vi "Type_0.vi"(7 "프런트패널 윈도우:동작":T1(ring)=enum."Default", 8 "에러 입력":errorcluster caption="에러 입력(에러 없음)", 11 "세부분류코드":string caption="확장자없는 파일 이름") -> (0 "error out":errorcluster)   [LabVIEW 2020]
uses:
  Support/Controls/Cmd_Mouse Popup.ctl
  Support/Controls/Clst_Query Info.ctl
  Support/Controls/Cmd_Read Query.ctl
  Support/Public/Polymorph/Array Dedup_1D Str.vi
  Support/Public/Polymorph/Cell Space_Table.vi
  <vilib>/addons/database/NI_Database_API.lvlib
panel:
  in  "탭 컨트롤":enum32{"검색", "등록", "CMC"}(tab)
  in  "일부추가":bool
  out "인정범위":string[][](table)
  out "SQL Quary 컬럼명":string
  out "Calfunc":string[][](array[string])
  out "모델정보":string[][](array[string])
  in  "옵션검색":bool
  in  "옵션 검색 조건":string(combo)
  in  "모델검색":bool
  in  "모델 검색 조건":string
  in  "측정범위검색":bool
  in  "범위 검색 조건":dbl
  in  "전체추가":bool
  out "소분류코드":string
  out "측정기명":string
  in  "최대 측정 범위":i32(listbox)
  in  "모델 및 옵션 List":i32(listbox)
  out "Load Proc":string[][](table) caption="등록된 교정 Procedure"
  in  "교정기능":string(combo)
  in  "구분 2":string(combo) caption="측정방향"
  in  "참고 버튼":bool
  in  "교정값":string
  in  "명목값":string caption="명목값 (호칭)"
  in  "추가단위":string(combo)="mg" caption="단위"
  in  "구분":string(combo) caption="측정위치"
  out "Func_ext ?":bool
  out "배열":u32[](array[numeric])
  in  "단위":string(combo)
  in  "변경 버튼":bool
  in  "등록 버튼":bool
  in  "교정점 추가 버튼":bool
  in  "교정점":string
  in  "Proc":string[][](table) caption="등록할 교정 Procedure"
  in  "형식":string
  in  "옵션":string
  in  "최소눈금":string(combo)
  in  "교정기능 2":string(combo) caption="세부기능"
  in  "표시방식":string(combo)
  out "CMC":string[][](table)
  # "항목정보"
  # "검색옵션"
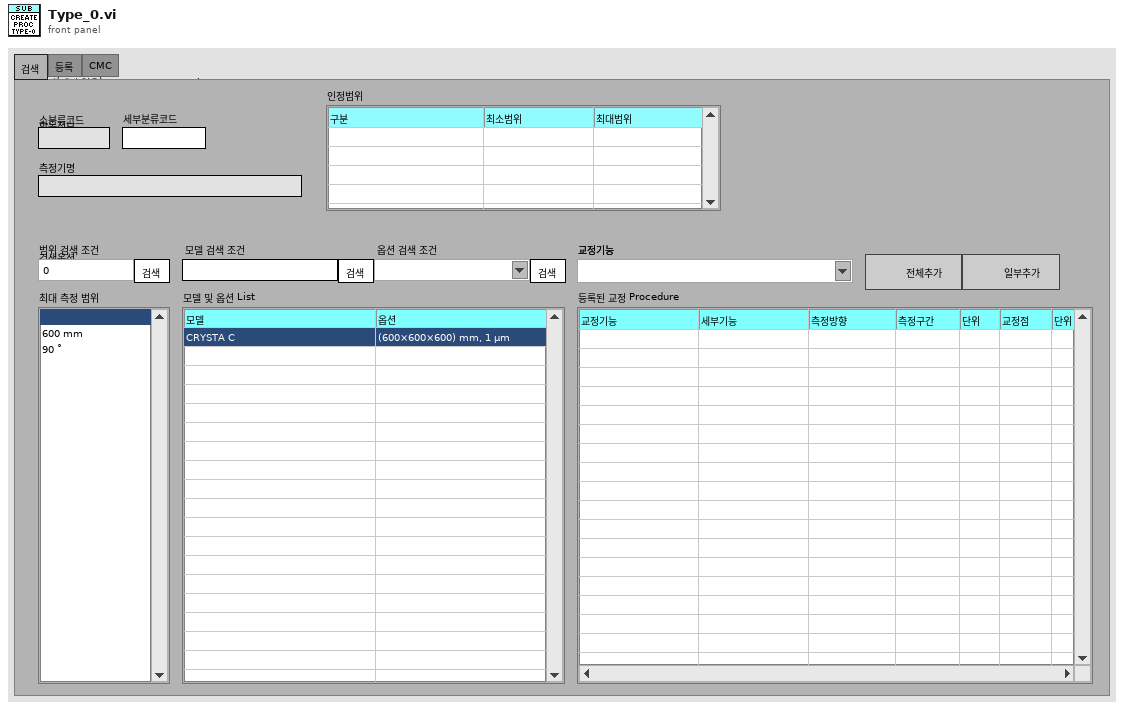
[diagram p1: front panel]
types:
  T1 = enum32{"Invalid", "Default", "Floating", "Floating/Auto-Hide", "Modal"}
  T2 = typedef "Cmd_Mouse Popup.ctl" = enum16{"활성화", "메뉴선택"}
  T3 = cluster{"Shift":bool, "Ctrl":bool, "Alt":bool, "Cmd":bool, "Opt":bool}
  T4 = typedef "Clst_Query Info.ctl" = cluster{"사번":string, "등록번호":string, "업체명":string, "세부분류코드":string, "형식":string, "기기번호":string, "FUNC":string, "FUNC_EXT":string, "옵션":string, "추가문자열":string, "일자":string, "배열 1":string[], "배열 2":string[], "항목명":string, "문자열":string, "이름":string}
  T5 = typedef "Cmd_Read Query.ctl" = enum16{"교정자 이름 얻기", "인증교정자 얻기", "기술책임자 얻기", "기책부책 얻기", "등록번호 얻기", "등록정보 얻기", "업체정보 얻기", "교정일자(CAMAS) 얻기", "교정일자(CALSTD) 얻기", "교정환경 얻기", "교정절차서 목록 얻기", "교정절차서명 얻기", "교정절차 목록얻기", "교정절차 얻기", "PROC 교정절차 얻기", "PROC SPEC 얻기", "교정절차(Func별) 얻기", "교정절차(Func_ext별) 얻기", "기관코드 얻기", "교정기능(세부분류) 얻기", "교정기능(모델) 얻기", "교정기능 목록 얻기", "교정기능 명칭 얻기", "교정기능 항목명칭 얻기", "DB (사용기준기) 얻기", "DB (기준기이름) 얻기", "DB (기준기이름목록) 얻기", "DB (기준기목록) 얻기", "DB (기준기값) 얻기", "DB (CMC) 얻기", "DB (FUNC) 얻기", "DB (CALNAME) 얻기", "DB (STDNAME) 얻기", "DB (SPEC) 얻기", "모델(항목전체) 얻기", "모델(최대범위) 얻기", "모델(최소범위) 얻기", "모델(최대최소) 얻기", "모델(범위조건) 얻기", "모델(등록요청) 얻기", "모델(형식별) 얻기", "모델(조건별) 얻기", "모델(모델검색) 얻기", "세부분류 목록 얻기", "기준기등록리스트 얻기", "STD Cal Date Check", "DB등록일자 얻기", "적용항목 얻기", "기타정보 얻기", "기준기요청 얻기", "서버버전 얻기"}
  T6 = cluster{refnum<vi>[], refnum<vi>[], refnum<vi>[], refnum<vi>[]}
  T7 = typedef "NI_Database_API.lvlib/Conn ObjectReference.ctl" = refnum<k1>
  T8 = typedef "LVRowAndColumnTypeDef.ctl" = cluster{"Row":i32, "Column":i32}
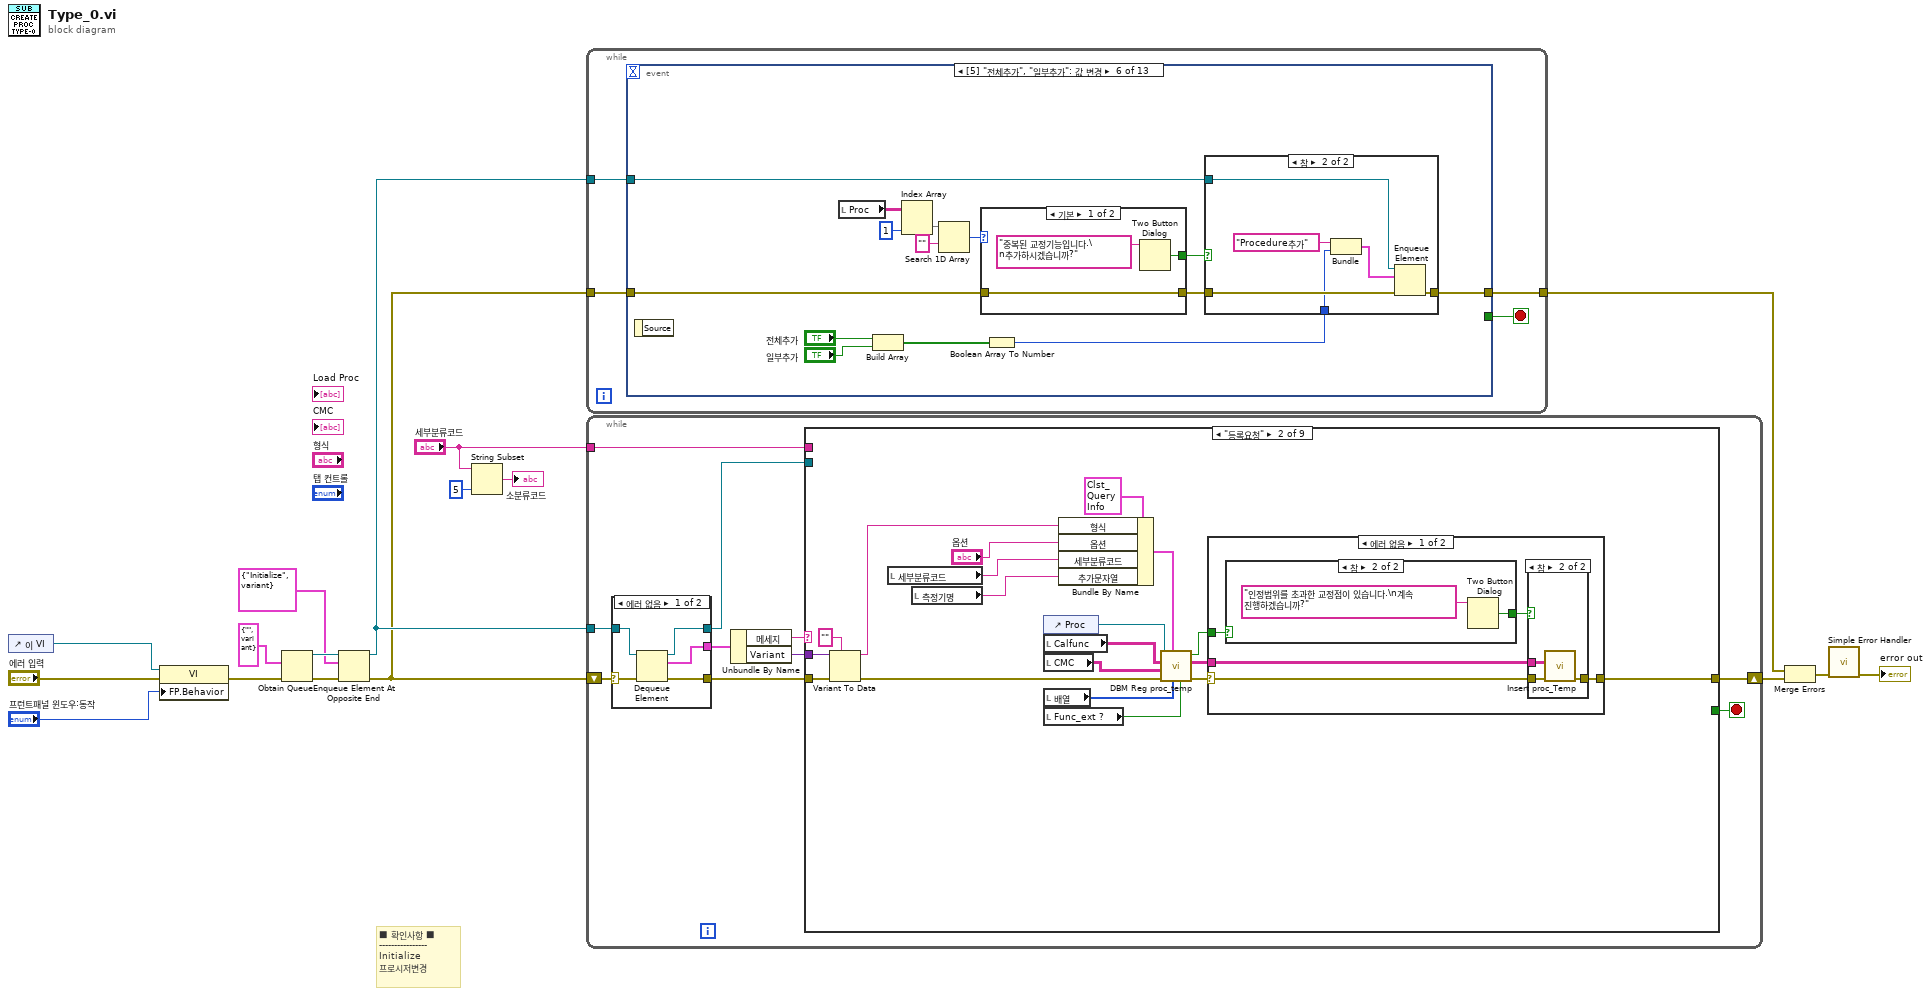
[diagram p0: block diagram]
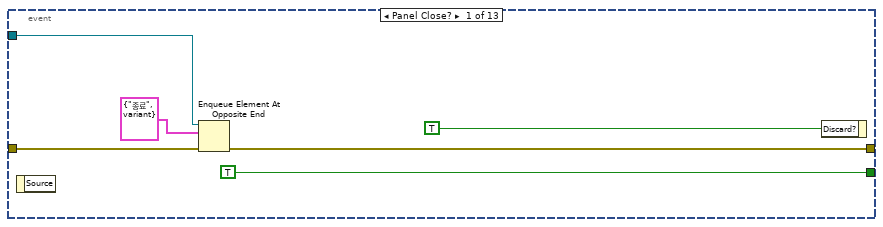
[diagram p2: hidden frame]
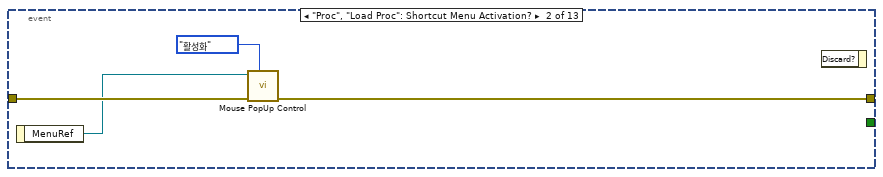
[diagram p3: hidden frame]
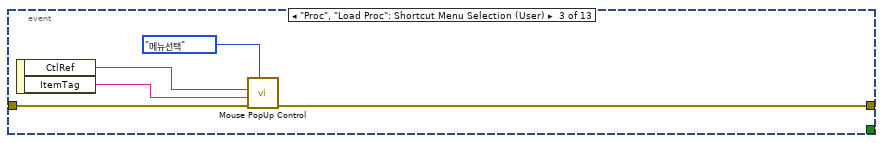
[diagram p4: hidden frame]
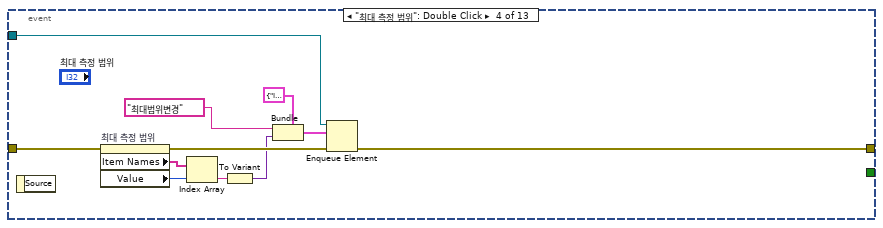
[diagram p5: hidden frame]
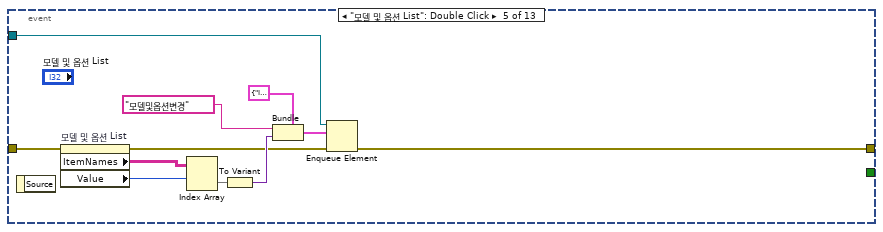
[diagram p6: hidden frame]
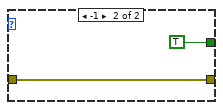
[diagram p8: hidden frame]
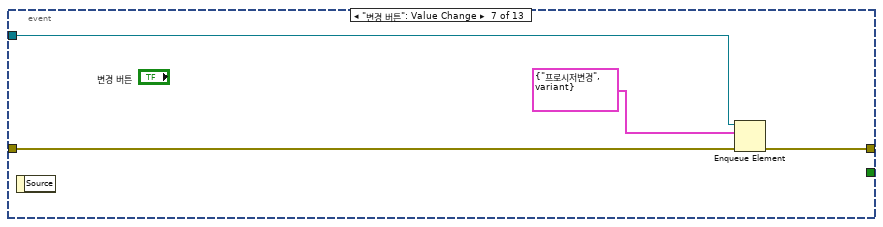
[diagram p9: hidden frame]
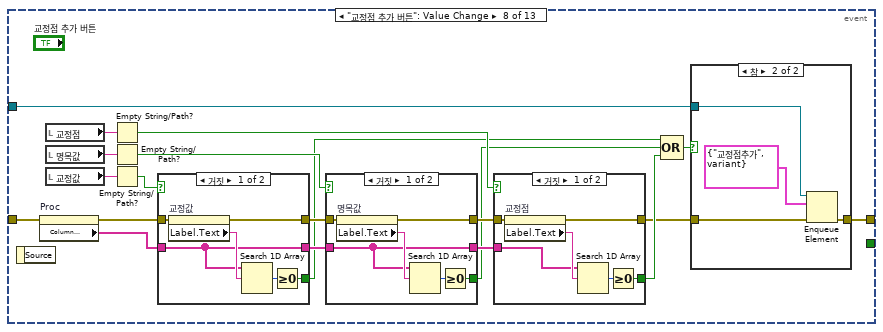
[diagram p10: hidden frame]
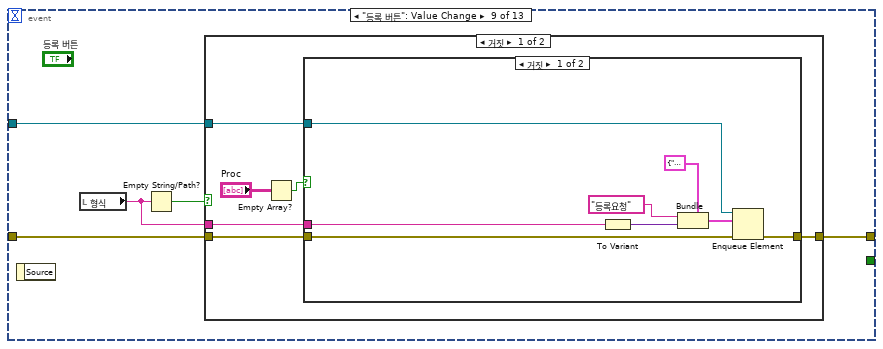
[diagram p15: hidden frame]
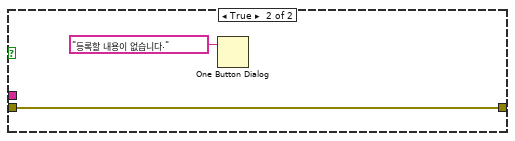
[diagram p16: hidden frame]
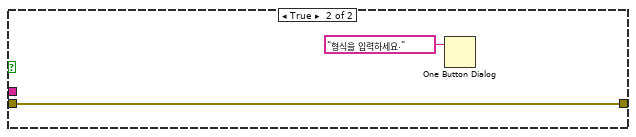
[diagram p17: hidden frame]
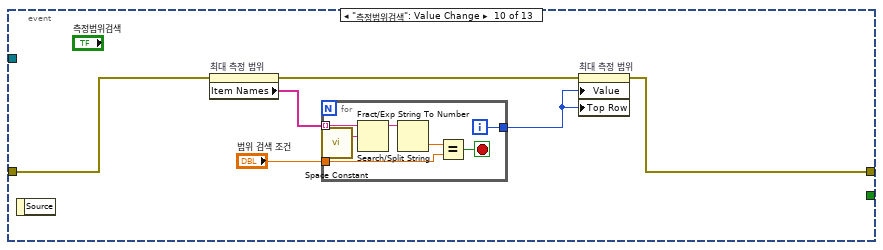
[diagram p18: hidden frame]
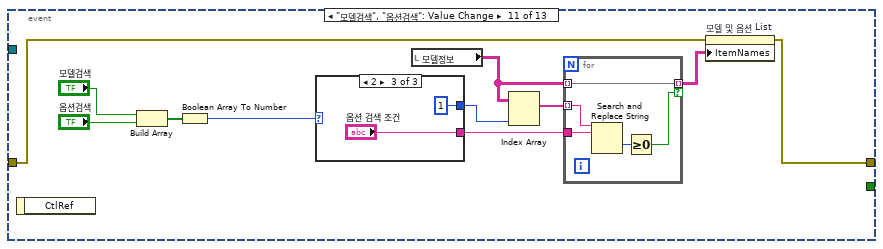
[diagram p19: hidden frame]
diagram:
  # "■ 확인사항 ■\n----------------\nInitialize\n프로시저변경"
  n1 = control-ref of="이 VI"() -> (w1:refnum<vi>)
  n2 = property class="VI"(reference=w1, error in="에러 입력", "FP.Behavior"="프런트패널 윈도우:동작") -> (error out=w7:errorcluster)  [unwired: 1 out]
  n3 = Obtain Queue(element data type=cluster{"메세지":string, "값":variant} {"메세지"="", "값"=variant} ("Message Cluster"), error in (no error)=w7) -> (queue out=w12:refnum<queue>, error out=w13:errorcluster)  [unwired: 3 in, 1 out]
  n4 = Enqueue Element At Opposite End(queue=w12, element=cluster{"메세지":string, "값":variant} {"메세지"="Initialize", "값"=variant} ("Message Cluster"), error in (no error)=w13) -> (queue out=w10:refnum<queue>, error out=w9:errorcluster)  [unwired: 1 in, 1 out]
  n5 = String Subset(string="세부분류코드", length (rest)=5 ("길이(나머지)")) -> (substring=→"소분류코드":string)  [unwired: 1 in]
  n6 = while {
    tunnel: w10 -> [w21]
    tunnel: w9 -> [w20]
    tunnel: [w19] -> w16
    stop <- w18 stop-if-true
    n7 = event shown="[5] \"전체추가\", \"일부추가\": 값 변경" {
      selector: _ -> [_ _ _ _ _ _ _ _ _ _ _ _ _]
      dyn-events: _ -> [_ _ _ _ _ _ _ _ _ _ _ _ _]
      timeout: _ -> [_ _ _ _ _ _ _ _ _ _ _ _ _]
      tunnel: w21 -> [w23 _ _ w46 w57 w71 w87 w107 w139 _ _ _ _]
      tunnel: w20 -> [w25 w31 w36 w45 w51 w70 w86 w106 w141 w165 w174 w198 _]
      tunnel: [w24 w30 w35 w47 w58 w72 w88 w108 w140 w162 w179 w197 _] -> w19
      tunnel: [TRUE ("우선순위 메시지?") _ _ _ _ _ _ _ _ _ _ _ _] -> w18
      event Panel Close? {
        n8 = event-data() -> ()  [unwired: 1 in, 1 out]
        n9 = Enqueue Element At Opposite End(queue=w23, element=cluster{"메세지":string, "값":variant} {"메세지"="종료", "값"=variant} ("원소"), error in (no error)=w25) -> (error out=w24:errorcluster)  [unwired: 1 in, 2 out]
        n10 = event-data("Discard?"=TRUE ("버림?")) -> ()  [unwired: 1 in, 1 out]
      }
      event "Proc", "Load Proc": Shortcut Menu Activation? {
        n11 = event-data() -> ("MenuRef"=w28:refnum<k9>)  [unwired: 1 in]
        n12 = call "Mouse PopUp Control.vi"("type"=Cmd_Mouse_Popup."활성화", "error in"=w31, "메뉴 참조"=w28) -> ("error out"=w30:errorcluster)  [unwired: 8 in]
        n13 = event-data() -> ()  [unwired: 2 in, 1 out]
      }
      event "Proc", "Load Proc": Shortcut Menu Selection (User) {
        n14 = event-data() -> ("CtlRef"=w32:refnum<vi>, "ItemTag"=w33:string)  [unwired: 1 in]
        n15 = call "Mouse PopUp Control.vi"("type"=Cmd_Mouse_Popup."메뉴선택", "error in"=w36, "아이템 태그"=w33, "Tbl 참조 번호"=w32) -> ("error out"=w35:errorcluster)  [unwired: 7 in]
      }
      event "최대 측정 범위": Double Click {
        n16 = event-data() -> ()  [unwired: 1 in, 1 out]
        n17 = property on="최대 측정 범위" class="LstBox (엄격한)"(error in=w45) -> (error out=w44:errorcluster, "Item Names"=w41:string[], "Value"=w40:i32)  [unwired: 1 in, 1 out]
        n18 = Index Array(array=w41, index=w40) -> (element=w39:string)
        n19 = To Variant(anything=w39) -> (Variant=w38:variant)
        n20 = Bundle(cluster=cluster{"메세지":string, "값":variant} {"메세지"="Initialize", "값"=variant} ("Message Cluster"), "메세지"="최대범위변경", "값"=w38) -> (w37:cluster{"메세지":string, "값":variant})
        n21 = Enqueue Element(queue=w46, element=w37, error in (no error)=w44) -> (error out=w47:errorcluster)  [unwired: 1 in, 2 out]
      }
      event "모델 및 옵션 List": Double Click {
        n22 = event-data() -> ()  [unwired: 1 in, 1 out]
        n23 = property on="모델 및 옵션 List" class="MCListbox (엄격한)"(error in=w51) -> (error out=w50:errorcluster, "ItemNames"=w49:string[][], "Value"=w48:i32)  [unwired: 1 in, 1 out]
        n24 = Index Array(array=w49, index (row)=w48) -> (element=w54:string[])  [unwired: 1 in]
        n25 = To Variant(anything=w54) -> (Variant=w53:variant)
        n26 = Bundle(cluster=cluster{"메세지":string, "값":variant} {"메세지"="Initialize", "값"=variant} ("Message Cluster"), "메세지"="모델및옵션변경", "값"=w53) -> (w52:cluster{"메세지":string, "값":variant})
        n27 = Enqueue Element(queue=w57, element=w52, error in (no error)=w50) -> (error out=w58:errorcluster)  [unwired: 1 in, 2 out]
      }
      event "전체추가", "일부추가": Value Change {
        n28 = event-data() -> ()  [unwired: 1 in, 1 out]
        n29 = local read "Proc"() -> (w67:string[][])
        n30 = Build Array("전체추가", "일부추가") -> (w60:bool[])
        n31 = Index Array(array=w67, index (col)=1 ("비활성화된 인덱스 (열)")) -> (element=w69:string[])  [unwired: 1 in]
        n32 = Search 1D Array(1D array=w69, element="" ("원소")) -> (index of element=w66:i32)  [unwired: 1 in]
        n33 = case shown="기본" w66 {
          tunnel: [w82 w83] -> w65
          tunnel: w70 -> [w82 w83]
          tunnel: [w80 TRUE ("T button?")] -> w64
          frame Default {
            n34 = Two Button Dialog(message="중복된 교정기능입니다.\n추가하시겠습니까?" ("메시지")) -> (T button?=w80:bool)  [unwired: 2 in]
          }
          frame -1 {
          }
        }
        n35 = Boolean Array To Number(Boolean array=w60) -> (number=w59:u32)
        n36 = case shown="참" w64 {
          tunnel: w71 -> [_ w79]
          tunnel: w65 -> [w73 w78]
          tunnel: [w73 w77] -> w72
          tunnel: w59 -> [_ w75]
          frame False {
          }
          frame True {
            n37 = Bundle("메세지"="Procedure추가", w75) -> (w74:cluster{"메세지":string, u32})  [unwired: 1 in]
            n38 = Enqueue Element(queue=w79, element=w74, error in (no error)=w78) -> (error out=w77:errorcluster)  [unwired: 1 in, 2 out]
          }
        }
      }
      event "변경 버튼": Value Change {
        n39 = event-data() -> ()  [unwired: 1 in, 1 out]
        n40 = Enqueue Element(queue=w87, element=cluster{"메세지":string, "값":variant} {"메세지"="프로시저변경", "값"=variant} ("Message Cluster"), error in (no error)=w86) -> (error out=w88:errorcluster)  [unwired: 1 in, 2 out]
      }
      event "교정점 추가 버튼": Value Change {
        n41 = event-data() -> ()  [unwired: 1 in, 1 out]
        n42 = property on="Proc" class="Tbl (엄격한)"(error in=w106) -> (error out=w96:errorcluster, "Column Headers[]"=w95:string[])  [unwired: 1 in, 1 out]
        n43 = local read "교정점"() -> (w105:string)
        n44 = local read "명목값"() -> (w102:string)
        n45 = local read "교정값"() -> (w101:string)
        n46 = Empty String/Path?(string/path=w105) -> (empty?=w100:bool)
        n47 = Empty String/Path?(string/path=w102) -> (empty?=w92:bool)
        n48 = Empty String/Path?(string/path=w101) -> (empty?=w91:bool)
        n49 = case shown="거짓" w91 {
          tunnel: [w114 w116] -> w99
          tunnel: w95 -> [w109 w115]
          tunnel: [w111 _] -> w90
          tunnel: w96 -> [w110 w116]
          tunnel: [w109 w115] -> w94
          frame False {
            n50 = property on="교정값" class="Str"(error in=w110) -> (error out=w114:errorcluster, "Label.Text"=w112:string)  [unwired: 1 in, 1 out]
            n51 = Search 1D Array(1D array=w109, element=w112) -> (index of element=w113:i32)  [unwired: 1 in]
            n52 = Greater Or Equal To 0?(x=w113) -> (x >= 0?=w111:bool)
          }
          frame True {
          }
        }
        n53 = case shown="거짓" w92 {
          tunnel: [w122 w124] -> w97
          tunnel: w94 -> [w117 w123]
          tunnel: [w119 _] -> w89
          tunnel: w99 -> [w118 w124]
          tunnel: [w117 w123] -> w93
          frame False {
            n54 = property on="명목값" class="Str"(error in=w118) -> (error out=w122:errorcluster, "Label.Text"=w120:string)  [unwired: 1 in, 1 out]
            n55 = Search 1D Array(1D array=w117, element=w120) -> (index of element=w121:i32)  [unwired: 1 in]
            n56 = Greater Or Equal To 0?(x=w121) -> (x >= 0?=w119:bool)
          }
          frame True {
          }
        }
        n57 = case shown="거짓" w100 {
          tunnel: [w130 w131] -> w98
          tunnel: w93 -> [w127 _]
          tunnel: [w126 _] -> w104
          tunnel: w97 -> [w125 w131]
          frame False {
            n58 = property on="교정점" class="Str"(error in=w125) -> (error out=w130:errorcluster, "Label.Text"=w128:string)  [unwired: 1 in, 1 out]
            n59 = Search 1D Array(1D array=w127, element=w128) -> (index of element=w129:i32)  [unwired: 1 in]
            n60 = Greater Or Equal To 0?(x=w129) -> (x >= 0?=w126:bool)
          }
          frame True {
          }
        }
        n61 = Compound Arithmetic op=OR(w90, w89, w104) -> (w103:bool)
        n62 = case shown="참" w103 {
          tunnel: [w132 w136] -> w108
          tunnel: w107 -> [_ w135]
          tunnel: w98 -> [w132 w133]
          frame False {
          }
          frame True {
            n63 = Enqueue Element(queue=w135, element=cluster{"메세지":string, "값":variant} {"메세지"="교정점추가", "값"=variant} ("Message Cluster"), error in (no error)=w133) -> (error out=w136:errorcluster)  [unwired: 1 in, 2 out]
          }
        }
      }
      event "등록 버튼": Value Change {
        n64 = event-data() -> ()  [unwired: 1 in, 1 out]
        n65 = local read "형식"() -> (w137:string)
        n66 = Empty String/Path?(string/path=w137) -> (empty?=w138:bool)
        n67 = case shown="거짓" w138 {
          tunnel: w141 -> [w147 w159]
          tunnel: [w146 w159] -> w140
          tunnel: w139 -> [w145 _]
          tunnel: w137 -> [w144 _]
          frame False {
            n68 = Empty Array?(array="Proc") -> (empty?=w143:bool)
            n69 = case shown="거짓" w143 {
              tunnel: w147 -> [w155 w157]
              tunnel: [w154 w157] -> w146
              tunnel: w145 -> [w153 _]
              tunnel: w144 -> [w152 _]
              frame False {
                n70 = To Variant(anything=w152) -> (Variant=w149:variant)
                n71 = Bundle(cluster=cluster{"메세지":string, "값":variant} {"메세지"="", "값"=variant} ("원소"), "메세지"="등록요청", "값"=w149) -> (w150:cluster{"메세지":string, "값":variant})
                n72 = Enqueue Element(queue=w153, element=w150, error in (no error)=w155) -> (error out=w154:errorcluster)  [unwired: 1 in, 2 out]
              }
              frame True {
                n73 = One Button Dialog(message="등록할 내용이 없습니다." ("메시지")) -> ()  [unwired: 1 in, 1 out]
              }
            }
          }
          frame True {
            n74 = One Button Dialog(message="형식을 입력하세요." ("메시지")) -> ()  [unwired: 1 in, 1 out]
          }
        }
      }
      event "측정범위검색": Value Change {
        n75 = event-data() -> ()  [unwired: 1 in, 1 out]
        n76 = property on="최대 측정 범위" class="LstBox (엄격한)"(error in=w165) -> (error out=w163:errorcluster, "Item Names"=w164:string[])  [unwired: 1 in, 1 out]
        n77 = for {
          tunnel: w164 -> [w171] mode=indexing
          tunnel: "범위 검색 조건" -> [w167]
          tunnel: [w172] -> w161
          i -> [w172]
          stop <- w166 stop-if-true
          n78 = call <vilib>:"Space Constant.vi"() -> ("String"=w170:string)
          n79 = Search/Split String(string=w171, search string/char (-)=w170) -> (substring before match=w169:string)  [unwired: 1 in, 2 out]
          n80 = Fract/Exp String To Number(string=w169) -> (number=w168:dbl)  [unwired: 3 in, 1 out]
          n81 = Equal?(x=w168, y=w167) -> (x = y?=w166:bool)
        }
        n82 = property on="최대 측정 범위" class="LstBox (엄격한)"(error in=w163, "Value"=w161, "Top Row"=w161) -> (error out=w162:errorcluster)  [unwired: 1 in, 1 out]
      }
      event "모델검색", "옵션검색": Value Change {
        n83 = event-data() -> ()  [unwired: 1 in, 1 out]
        n84 = Build Array("모델검색", "옵션검색") -> (w177:bool[])
        n85 = Boolean Array To Number(Boolean array=w177) -> (number=w175:u32)
        n86 = case shown="2" w175 {
          tunnel: [_ 0 ("비활성화된 인덱스 (열)") 1 ("비활성화된 인덱스 (열)")] -> w182
          tunnel: [_ "모델 검색 조건" "옵션 검색 조건"] -> w181
          frame Default {
          }
          frame 1 {
          }
          frame 2 {
          }
        }
        n87 = local read "모델정보"() -> (w173:string[][])
        n88 = Index Array(array=w173, index (col)=w182) -> (element=w183:string[])  [unwired: 1 in]
        n89 = for {
          tunnel: w183 -> [w192] mode=indexing
          tunnel: w181 -> [w191]
          tunnel: w173 -> [w189] mode=indexing
          tunnel: [w189] -> w180 mode=indexing if=w188
          n90 = Search and Replace String(input string=w192, search string=w191) -> (offset past replacement=w190:i32)  [unwired: 6 in, 3 out]
          n91 = Greater Or Equal To 0?(x=w190) -> (x >= 0?=w188:bool)
        }
        n92 = property on="모델 및 옵션 List" class="MCListbox (엄격한)"(error in=w174, "ItemNames"=w180) -> (error out=w179:errorcluster)  [unwired: 1 in, 1 out]
      }
      event "Proc": Key Down; "Proc": Key Repeat {
        n93 = event-data() -> ("PlatMods"=w193:T3, "ScanCode"=w196:i16, "Mods.Num Pad"=w195:bool, "CtlRef"=w194:refnum<vi>)  [unwired: 1 in]
        n94 = call "Cursor Control.vi"("플랫폼 조합키"=w193, "참조"=w194, "Num Pad"=w195, "ScanCode"=w196, "error in"=w198) -> ("error out"=w197:errorcluster)  [unwired: 5 in, 1 out]
      }
      event "참고 버튼": Value Change {
        n95 = event-data() -> ()  [unwired: 1 in, 1 out]
        n96 = call "DBM Reference.vi"() -> ()  [unwired: 12 in]
      }
    }
  }
  n97 = while {
    tunnel: w10 -> [w207]
    shift-right: [w199] -> w17
    shift-left: w9 -> [w203]
    tunnel: "세부분류코드" -> [w200]
    stop <- w208 stop-if-true
    n98 = case shown="에러 없음" w203 {
      selector: w203 -> [w209 w214]
      tunnel: w207 -> [w213 w218]
      tunnel: [w212 _] -> w201
      tunnel: [w210 w218] -> w206
      tunnel: [w211 w217] -> w202
      frame No Error {
        n99 = Dequeue Element(queue=w213, error in (no error)=w209) -> (queue out=w210:refnum<queue>, element=w211:cluster{"메세지":string, "값":variant}, error out=w212:errorcluster)  [unwired: 1 in, 1 out]
      }
      frame Error {
        n100 = To Variant(anything=w214) -> (Variant=w215:variant)
        n101 = Bundle("에러", "Variant"=w215) -> (w217:cluster{string, "Variant":variant})  [unwired: 1 in]
      }
    }
    n102 = Unbundle By Name(w202) -> ("메세지"=w204:string, "Variant"=w205:variant)
    n103 = case shown="\"등록요청\"" w204 {
      tunnel: w201 -> [w256 w289 w318 w343 w353 w398 w571 w716 w721]
      tunnel: w206 -> [_ _ _ _ _ _ _ _ _]
      tunnel: w205 -> [_ w288 w317 w342 w352 _ _ _ w719]
      tunnel: [_ _ _ _ _ _ _ TRUE _] -> w208
      tunnel: w200 -> [w223 _ _ _ _ _ w559 _ _]
      tunnel: [w250 w275 w313 w338 w356 w387 w569 w716 w718] -> w199
      frame "Initialize", Default {
        w246 = ""
        w257 = TRUE ("정렬?")
        w268 = string[][] [] ("Proc")
        n104 = control-ref of="모델 및 옵션 List"() -> (w271:refnum<vi>)
        n105 = control-ref of="CMC"() -> (w230:refnum<vi>)
        n106 = local write "교정기능 2"(w246) -> ()
        n107 = local write "최소눈금"(w246) -> ()
        n108 = local write "표시방식"(w246) -> ()
        n109 = local write "단위"(w246) -> ()
        n110 = local write "교정점"(w246) -> ()
        n111 = local write "명목값"(w246) -> ()
        n112 = local write "교정값"(w246) -> ()
        n113 = local write "추가단위"(w246) -> ()
        n114 = local write "탭 컨트롤"(enum32{"검색", "등록", "CMC"}."검색" ("탭 컨트롤")) -> ()
        n115 = local write "Proc"(w268) -> ()
        n116 = local write "Load Proc"(w268) -> ()
        n117 = Build Array(w271) -> (w266:refnum<vi>[])
        n118 = call "Start Create Procedure.vi"("에러 입력(에러 없음)"=w256, "Model List"=w266, "세부분류코드"=w223, "CMC"=w230) -> ("에러 출력"=w239:errorcluster, "Calfunc"=w221:string[][], "CMC"=→"인정범위":string[][], "모델정보 배열"=w219:string[][], "모델 및 옵션"=→"모델정보":string[][])  [unwired: 2 in, 1 out]
        "Calfunc" <- w221
        n119 = Index Array(array=w219, index (col) #1=1 ("비활성화된 인덱스 (열)"), index (col) #2=5 ("비활성화된 인덱스 (열)")) -> (element #1=w259:string[], element #2=w269:string[])  [unwired: 2 in]
        n120 = call-poly "Array Deduplication.vi"("정렬?"=w257, "배열 in"=w259) -> ("배열 out"=w258:string[])  [unwired: 8 in, 1 out]
        n121 = call-poly "Array Deduplication.vi"("정렬?"=w257, "배열 in"=w269) -> ("배열 out"=w265:string[])  [unwired: 8 in, 1 out]
        n122 = Index Array(array=w221, index (row) #1=0 ("인덱스 (열)"), index (col) #1=4 ("비활성화된 인덱스 (열)"), index (col) #2=3 ("비활성화된 인덱스 (열)")) -> (element #1=→"측정기명":string, element #2=w228:string[])  [unwired: 1 in]
        n123 = property on="옵션 검색 조건" class="CmbBox"(error in=w239, "Strings[]"=w258) -> (error out=w260:errorcluster)  [unwired: 1 in, 1 out]
        n124 = control-ref of="표시방식"() -> (w254:refnum<vi>)
        n125 = control-ref of="단위"() -> (w255:refnum<vi>)
        n126 = control-ref of="추가단위"() -> (w245:refnum<vi>)
        n127 = Insert Into Array(array=w265, index=0 ("인덱스"), new element="") -> (w263:string[])
        n128 = property on="최대 측정 범위" class="LstBox (엄격한)"(error in=w260, "Item Names"=w263) -> (error out=w236:errorcluster)  [unwired: 1 in, 1 out]
        n129 = control-ref of="추가단위"() -> (w244:refnum<vi>)
        n130 = control-ref of="교정기능 2"() -> (w240:refnum<vi>)
        n131 = control-ref of="최소눈금"() -> (w249:refnum<vi>)
        n132 = control-ref of="표시방식"() -> (w248:refnum<vi>)
        n133 = control-ref of="단위"() -> (w247:refnum<vi>)
        n134 = control-ref of="구분"() -> (w238:refnum<vi>)
        n135 = control-ref of="구분 2"() -> (w237:refnum<vi>)
        n136 = control-ref of="교정점"() -> (w241:refnum<vi>)
        n137 = control-ref of="명목값"() -> (w242:refnum<vi>)
        n138 = control-ref of="교정값"() -> (w243:refnum<vi>)
        n139 = Build Array(w254, w255, w245) -> (w227:refnum<vi>[])
        n140 = control-ref of="Proc"() -> (w253:refnum<vi>)
        n141 = control-ref of="Load Proc"() -> (w252:refnum<vi>)
        n142 = Build Array(w241, w242, w243, w244) -> (w225:refnum<vi>[])
        n143 = Build Array(w240, w249, w248, w247, w238, w237) -> (w224:refnum<vi>[])
        n144 = Build Array(w253, w252) -> (w226:refnum<vi>[])
        n145 = property on="교정기능" class="CmbBox"(error in=w236, "Strings[]"=w228) -> (error out=w235:errorcluster)  [unwired: 1 in, 1 out]
        n146 = Bundle(w227, w226, w225, w224) -> (w222:T6)  [unwired: 1 in]
        n147 = call "DBM Unit Set.vi"("분류코드"=w223, "에러 입력(에러 없음)"=w235, "교정기능 문자열[]"=w228, "참조"=w222) -> ("에러 출력"=w250:errorcluster, "SQL query 컬럼명"=→"SQL Quary 컬럼명":string)  [unwired: 5 in, 1 out]
      }
      frame "등록요청" {
        n148 = Variant To Data(error in=w289, type="", Variant=w288) -> (data=w285:string)  [unwired: 1 out]
        n149 = local read "세부분류코드"() -> (w283:string)
        n150 = local read "측정기명"() -> (w282:string)
        n151 = control-ref of="Proc"() -> (w276:refnum<vi>)
        n152 = local read "Calfunc"() -> (w280:string[][])
        n153 = local read "CMC"() -> (w281:string[][])
        n154 = local read "배열"() -> (w279:u32[])
        n155 = local read "Func_ext ?"() -> (w278:bool)
        n156 = Bundle By Name(cluster=T4 {"사번"="", "등록번호"="", "업체명"="", "세부분류코드"="", "형식"="", "기기번호"="", "FUNC"="", "FUNC_EXT"="", "옵션"="", "추가문자열"="", "일자"="", "배열 1"=[], "배열 2"=[], "항목명"="", "문자열"="", "이름"=""} ("Query info"), "형식"=w285, "옵션"="옵션", "세부분류코드"=w283, "추가문자열"=w282) -> (w277:T4)
        n157 = call "DBM Reg proc_temp.vi"("Calfunc ?"=w278, "배열"=w279, "Query info"=w277, "에러 입력"=w289, "CMC"=w281, "calfunc"=w280, "Proc 참조 in"=w276) -> ("에러 출력"=w274:errorcluster, "배열출력"=w273:string[][], "에러?"=w272:bool)  [unwired: 2 in]
        n158 = case shown="에러 없음" w274 {
          selector: w274 -> [w290 w302]
          tunnel: w272 -> [w294 _]
          tunnel: [w293 w302] -> w275
          tunnel: w273 -> [w292 _]
          frame No Error {
            n159 = case shown="참" w294 {
              tunnel: [TRUE ("T button?") w296] -> w291
              frame False {
              }
              frame True {
                n160 = Two Button Dialog(message="인정범위를 초과한 교정점이 있습니다.\n계속 진행하겠습니까?" ("메시지")) -> (T button?=w296:bool)  [unwired: 2 in]
              }
            }
            n161 = case shown="참" w291 {
              tunnel: [w298 w301] -> w293
              tunnel: w290 -> [w298 w300]
              tunnel: w292 -> [_ w299]
              frame False {
              }
              frame True {
                n162 = call "Insert proc_Temp.vi"("에러 입력(에러 없음)"=w300, "Proc 입력"=w299) -> ("에러 출력"=w301:errorcluster)  [unwired: 9 in]
              }
            }
          }
          frame Error {
          }
        }
      }
      frame "최대범위변경" {
        n163 = local read "세부분류코드"() -> (w303:string)
        n164 = Variant To Data(error in=w318, type="", Variant=w317) -> (data=w305:string, error out=w316:errorcluster)
        n165 = call "DB Open.vi"("에러 입력"=w316) -> ("에러 출력"=w312:errorcluster, "참조 번호 출력"=w309:T7)  [unwired: 9 in]
        n166 = Bundle By Name(cluster=T4 {"사번"="", "등록번호"="", "업체명"="", "세부분류코드"="", "형식"="", "기기번호"="", "FUNC"="", "FUNC_EXT"="", "옵션"="", "추가문자열"="", "일자"="", "배열 1"=[], "배열 2"=[], "항목명"="", "문자열"="", "이름"=""} ("Query info"), "세부분류코드"=w303, "추가문자열"=w305) -> (w304:T4)
        n167 = call "DB Read Queries.vi"("Query info"=w304, "Query Command"=Cmd_Read_Query."모델(최대범위) 얻기", "에러 입력(에러 없음)"=w312, "참조 번호 입력"=w309) -> ("에러 출력"=w311:errorcluster, "Data"=w310:string[][], "참조 번호 출력"=w308:T7)  [unwired: 3 in, 2 out]
        n168 = call <vilib>:"DB Tools Close Connection.vi"("error in (no error)"=w311, "connection reference"=w308) -> ("error out"=w314:errorcluster)  [unwired: 5 in]
        n169 = property on="모델 및 옵션 List" class="MCListbox (엄격한)"(error in=w314, "ItemNames"=w310) -> (error out=w313:errorcluster)  [unwired: 1 in, 1 out]
      }
      frame "모델및옵션변경" {
        n170 = local read "세부분류코드"() -> (w330:string)
        n171 = Variant To Data(error in=w343, type=string[] [], Variant=w342) -> (data=w339:string[], error out=w341:errorcluster)
        n172 = Index Array(array=w339) -> (element #1=w329:string, element #2=w328:string)  [unwired: 2 in]
        n173 = Bundle By Name(cluster=T4 {"사번"="", "등록번호"="", "업체명"="", "세부분류코드"="", "형식"="", "기기번호"="", "FUNC"="", "FUNC_EXT"="", "옵션"="", "추가문자열"="", "일자"="", "배열 1"=[], "배열 2"=[], "항목명"="", "문자열"="", "이름"=""} ("Query info"), "세부분류코드"=w330, "형식"=w329, "옵션"=w328) -> (w327:T4)
        n174 = call "DB Open.vi"("에러 입력"=w341) -> ("에러 출력"=w336:errorcluster, "참조 번호 출력"=w334:T7)  [unwired: 9 in]
        n175 = local read "SQL Quary 컬럼명"() -> (w319:string)
        n176 = call "DB Read Queries.vi"("Query info"=w327, "Query Command"=Cmd_Read_Query."교정절차 얻기", "에러 입력(에러 없음)"=w336, "참조 번호 입력"=w334) -> ("에러 출력"=w335:errorcluster, "Data"=w326:string[][], "참조 번호 출력"=w333:T7)  [unwired: 3 in, 2 out]
        n177 = call <vilib>:"DB Tools Close Connection.vi"("error in (no error)"=w335, "connection reference"=w333) -> ("error out"=w324:errorcluster)  [unwired: 5 in]
        n178 = local read "Calfunc"() -> (w320:string[][])
        n179 = call "Condition Filter.vi"("Cal func in"=w320, "컬럼명"=w319, "error in (no error)"=w324, "Cal Proc in"=w326) -> ("error out"=w323:errorcluster, "배열"=→"배열":u32[], "Func_ext ?"=→"Func_ext ?":bool, "Cal Proc out"=w325:string[][])  [unwired: 4 in]
        n180 = control-ref of="Load Proc"() -> (w337:refnum<vi>)
        n181 = call-poly "Cell Spacing.vi"("error in"=w323, "Data in"=w325, "테이블 참조 in"=w337) -> ("error out"=w338:errorcluster)  [unwired: 6 in, 2 out]
      }
      frame "Procedure추가" {
        n182 = Variant To Data(error in=w353, type=u32 0 ("숫자"), Variant=w352) -> (data=w349:u32, error out=w351:errorcluster)
        n183 = local read "Load Proc"() -> (w357:string[][])
        n184 = Empty String/Path?(string/path="교정기능") -> (empty?=w347:bool)
        n185 = local read "Func_ext ?"() -> (w345:bool)
        n186 = Not(x=w345) -> (.not. x?=w344:bool)
        n187 = Or(x=w347, y=w344) -> (x .or. y?=w346:bool)
        n188 = case shown="거짓" w346 {
          tunnel: [w362 w366] -> w360
          tunnel: w357 -> [w362 w365]
          tunnel: w349 -> [_ w364]
          tunnel: "교정기능" -> [_ w363]
          frame True {
          }
          frame False {
            n189 = case shown="1, 기본" w364 {
              tunnel: [w368 w374] -> w366
              tunnel: w365 -> [w369 w376]
              tunnel: w363 -> [w367 w375]
              frame 1, Default {
                n190 = for {
                  tunnel: w369 -> [w373] mode=indexing
                  tunnel: w367 -> [w370]
                  tunnel: [w372] -> w368 mode=indexing
                  n191 = Replace Array Subset(array=w373, new element=w370, index=1 ("인덱스")) -> (w372:string[])
                }
              }
              frame 2 {
                n192 = for {
                  tunnel: w376 -> [w381] mode=indexing
                  tunnel: w375 -> [w378]
                  tunnel: [w381] -> w374 mode=indexing if=w377
                  n193 = Index Array(array=w381, index=1 ("인덱스")) -> (element=w379:string)
                  n194 = Equal?(x=w379, y=w378) -> (x = y?=w377:bool)
                }
              }
            }
          }
        }
        n195 = local write "탭 컨트롤"(enum32{"검색", "등록", "CMC"}."등록" ("탭 컨트롤")) -> ()
        n196 = local read "Proc"() -> (w361:string[][])
        n197 = Empty Array?(array=w361) -> (empty?=w359:bool)
        n198 = case shown="거짓" w359 {
          tunnel: w361 -> [w384 _]
          tunnel: w360 -> [w383 w385]
          tunnel: [w382 w385] -> w354
          frame False {
            n199 = Insert Into Array(array=w384, new element=w383) -> (w382:string[][])  [unwired: 2 in]
          }
          frame True {
          }
        }
        n200 = control-ref of="Proc"() -> (w355:refnum<vi>)
        n201 = call-poly "Cell Spacing.vi"("error in"=w351, "Data in"=w354, "테이블 참조 in"=w355) -> ("error out"=w356:errorcluster)  [unwired: 6 in, 2 out]
      }
      frame "프로시저변경" {
        n202 = property on="Proc" class="Tbl (엄격한)"(error in=w398) -> (error out=w386:errorcluster, "Selection Size"=w396:T8, "Selection Start"=w397:T8)  [unwired: 1 in, 1 out]
        n203 = local read "Proc"() -> (w418:string[][])
        n204 = Unbundle By Name(w396) -> ("Row"=w393:i32)
        n205 = Unbundle By Name(w397) -> ("Row"=w395:i32)
        n206 = Add(x=w393, y=w395) -> (x+y=w394:i32)
        n207 = property on="Proc" class="Tbl (엄격한)"(error in=w386) -> (error out=w413:errorcluster, "Column Headers[]"=w390:string[])  [unwired: 1 in, 1 out]
        n208 = property on="최소눈금" class="CmbBox"(error in=w413) -> (error out=w410:errorcluster, "Label.Text"=w412:string)  [unwired: 1 in, 1 out]
        n209 = property on="단위" class="CmbBox"(error in=w410) -> (error out=w406:errorcluster, "Label.Text"=w409:string)  [unwired: 1 in, 1 out]
        n210 = Search 1D Array(1D array=w390, element=w412) -> (index of element=w411:i32)  [unwired: 1 in]
        n211 = Search 1D Array(1D array=w390, element=w409) -> (index of element=w408:i32)  [unwired: 1 in]
        n212 = Increment(x=w408) -> (x+1=w403:i32)
        n213 = property on="표시방식" class="CmbBox"(error in=w406) -> (error out=w401:errorcluster, "Label.Text"=w405:string)  [unwired: 1 in, 1 out]
        n214 = Search 1D Array(1D array=w390, element=w409, start index (0)=w403) -> (index of element=w407:i32)
        n215 = property on="구분" class="CmbBox"(error in=w401) -> (error out=w392:errorcluster, "Caption.Text"=w400:string)  [unwired: 1 in, 1 out]
        n216 = Search 1D Array(1D array=w390, element=w405) -> (index of element=w404:i32)  [unwired: 1 in]
        n217 = property on="구분 2" class="CmbBox"(error in=w392) -> (error out=w387:errorcluster, "Caption.Text"=w391:string)  [unwired: 1 in, 1 out]
        n218 = Search 1D Array(1D array=w390, element=w400) -> (index of element=w399:i32)  [unwired: 1 in]
        n219 = Search 1D Array(1D array=w390, element=w391) -> (index of element=w389:i32)  [unwired: 1 in]
        n220 = for {
          tunnel: w418 -> [w438] mode=indexing
          tunnel: "최소눈금" -> [w440]
          tunnel: [w439] -> w417 mode=indexing
          tunnel: "교정기능 2" -> [w436]
          tunnel: "단위" -> [w437]
          tunnel: "표시방식" -> [w435]
          tunnel: w411 -> [w434]
          tunnel: w408 -> [w433]
          tunnel: w407 -> [w432]
          tunnel: w404 -> [w431]
          tunnel: "구분" -> [w430]
          tunnel: w399 -> [w429]
          tunnel: w395 -> [w427]
          tunnel: w394 -> [w425]
          tunnel: w393 -> [w422]
          tunnel: w389 -> [w421]
          tunnel: "구분 2" -> [w420]
          i -> [w428]
          n221 = In Range and Coerce(upper limit=w425, x=w428, lower limit=w427) -> (In Range?=w426:bool)  [unwired: 1 out]
          n222 = Equal To 0?(x=w422) -> (x = 0?=w423:bool)
          n223 = Or(x=w423, y=w426) -> (x .or. y?=w424:bool)
          n224 = case shown="참" w424 {
            tunnel: w440 -> [_ w455]
            tunnel: [w441 w454] -> w439
            tunnel: w438 -> [w441 w453]
            tunnel: w437 -> [_ w452]
            tunnel: w436 -> [_ w451]
            tunnel: w435 -> [_ w450]
            tunnel: w434 -> [_ w449]
            tunnel: w433 -> [_ w448]
            tunnel: w432 -> [_ w447]
            tunnel: w431 -> [_ w446]
            tunnel: w430 -> [_ w445]
            tunnel: w429 -> [_ w444]
            tunnel: w421 -> [_ w443]
            tunnel: w420 -> [_ w442]
            frame False {
            }
            frame True {
              n225 = case shown="\"\"" w451 {
                selector: w451 -> [w469 _]
                tunnel: w455 -> [w467 w530]
                tunnel: [w471 w532] -> w454
                tunnel: w453 -> [w468 w531]
                tunnel: w452 -> [w466 w529]
                tunnel: w450 -> [w464 w528]
                tunnel: w449 -> [w463 w527]
                tunnel: w448 -> [w462 w526]
                tunnel: w447 -> [w461 w525]
                tunnel: w446 -> [w460 w524]
                tunnel: w445 -> [w459 w523]
                tunnel: w444 -> [w458 w522]
                tunnel: w443 -> [w457 w521]
                tunnel: w442 -> [w456 w520]
                frame Default {
                  n226 = Index Array(array=w468) -> (element #2=w470:string)  [unwired: 2 in, 1 out]
                  n227 = Equal?(x=w470, y=w469) -> (x = y?=w465:bool)
                  n228 = case shown="참" w465 {
                    tunnel: [w472 w475] -> w471
                    tunnel: w468 -> [w472 w489]
                    tunnel: w467 -> [_ w487]
                    tunnel: w466 -> [_ w486]
                    tunnel: w464 -> [_ w484]
                    tunnel: w463 -> [_ w483]
                    tunnel: w462 -> [_ w482]
                    tunnel: w461 -> [_ w481]
                    tunnel: w460 -> [_ w480]
                    tunnel: w459 -> [_ w478]
                    tunnel: w458 -> [_ w477]
                    tunnel: w457 -> [_ w474]
                    tunnel: w456 -> [_ w473]
                    frame False {
                    }
                    frame True {
                      n229 = case shown="기본" w487 {
                        selector: w487 -> [_ w507]
                        tunnel: [w505 w509] -> w488
                        tunnel: w489 -> [w505 w508]
                        tunnel: w483 -> [_ w506]
                        frame "" {
                        }
                        frame Default {
                          n230 = Replace Array Subset(array=w508, new element=w507, index=w506) -> (w509:string[])
                        }
                      }
                      n231 = case shown="기본" w486 {
                        selector: w486 -> [_ w513]
                        tunnel: [w510 w515] -> w485
                        tunnel: w488 -> [w510 w514]
                        tunnel: w482 -> [_ w512]
                        tunnel: w481 -> [_ w511]
                        frame "" {
                        }
                        frame Default {
                          n232 = Replace Array Subset(array=w514, new element #1=w513, index #1=w512, new element #2=w513, index #2=w511) -> (w515:string[])
                        }
                      }
                      n233 = case shown="기본" w484 {
                        selector: w484 -> [_ w502]
                        tunnel: [w500 w504] -> w479
                        tunnel: w485 -> [w500 w503]
                        tunnel: w480 -> [_ w501]
                        frame "" {
                        }
                        frame Default {
                          n234 = Replace Array Subset(array=w503, new element=w502, index=w501) -> (w504:string[])
                        }
                      }
                      n235 = case shown="기본" w478 {
                        selector: w478 -> [_ w497]
                        tunnel: [w495 w499] -> w476
                        tunnel: w479 -> [w495 w498]
                        tunnel: w477 -> [_ w496]
                        frame "" {
                        }
                        frame Default {
                          n236 = Replace Array Subset(array=w498, new element=w497, index=w496) -> (w499:string[])
                        }
                      }
                      n237 = case shown="기본" w473 {
                        selector: w473 -> [_ w492]
                        tunnel: [w490 w494] -> w475
                        tunnel: w476 -> [w490 w493]
                        tunnel: w474 -> [_ w491]
                        frame "" {
                        }
                        frame Default {
                          n238 = Replace Array Subset(array=w493, new element=w492, index=w491) -> (w494:string[])
                        }
                      }
                    }
                  }
                }
                frame "" {
                  n239 = case shown="\"\"" w530 {
                    selector: w530 -> [_ w550]
                    tunnel: [w548 w552] -> w519
                    tunnel: w531 -> [w548 w551]
                    tunnel: w527 -> [_ w549]
                    frame "" {
                    }
                    frame Default {
                      n240 = Replace Array Subset(array=w551, new element=w550, index=w549) -> (w552:string[])
                    }
                  }
                  n241 = case shown="\"\"" w529 {
                    selector: w529 -> [_ w556]
                    tunnel: [w553 w558] -> w518
                    tunnel: w519 -> [w553 w557]
                    tunnel: w526 -> [_ w555]
                    tunnel: w525 -> [_ w554]
                    frame "" {
                    }
                    frame Default {
                      n242 = Replace Array Subset(array=w557, new element #1=w556, index #1=w555, new element #2=w556, index #2=w554) -> (w558:string[])
                    }
                  }
                  n243 = case shown="기본" w528 {
                    selector: w528 -> [_ w545]
                    tunnel: [w543 w547] -> w517
                    tunnel: w518 -> [w543 w546]
                    tunnel: w524 -> [_ w544]
                    frame "" {
                    }
                    frame Default {
                      n244 = Replace Array Subset(array=w546, new element=w545, index=w544) -> (w547:string[])
                    }
                  }
                  n245 = case shown="\"\"" w523 {
                    selector: w523 -> [_ w540]
                    tunnel: [w538 w542] -> w516
                    tunnel: w517 -> [w538 w541]
                    tunnel: w522 -> [_ w539]
                    frame "" {
                    }
                    frame Default {
                      n246 = Replace Array Subset(array=w541, new element=w540, index=w539) -> (w542:string[])
                    }
                  }
                  n247 = case shown="\"\"" w520 {
                    selector: w520 -> [_ w535]
                    tunnel: [w533 w537] -> w532
                    tunnel: w516 -> [w533 w536]
                    tunnel: w521 -> [_ w534]
                    frame "" {
                    }
                    frame Default {
                      n248 = Replace Array Subset(array=w536, new element=w535, index=w534) -> (w537:string[])
                    }
                  }
                }
              }
            }
          }
        }
        n249 = local write "Proc"(w417) -> ()
      }
      frame "교정점추가" {
        w563 = "단위" ("원소")
        n250 = property on="Proc" class="Tbl (엄격한)"(error in=w571) -> (error out=w570:errorcluster, "Column Headers[]"=w564:string[], "Value"=w577:string[][], "Selection Start"=w578:T8)  [unwired: 1 in, 1 out]
        n251 = Unbundle(w578) -> ("Row"=w576:i32)  [unwired: 1 out]
        n252 = property on="교정점" class="Str"(error in=w570) -> (error out=w565:errorcluster, "Label.Text"=w575:string)  [unwired: 1 in, 1 out]
        n253 = Search 1D Array(1D array=w564, element=w575) -> (index of element=w568:i32)  [unwired: 1 in]
        n254 = Search 1D Array(1D array=w564, element=w563) -> (index of element=w562:i32)  [unwired: 1 in]
        n255 = Increment(x=w562) -> (x+1=w561:i32)
        n256 = Search 1D Array(1D array=w564, element=w563, start index (0)=w561) -> (index of element=w560:i32)
        n257 = property on="명목값" class="Str"(error in=w565) -> (error out=w573:errorcluster, "Label.Text"=w574:string)  [unwired: 1 in, 1 out]
        n258 = Search 1D Array(1D array=w564, element=w574) -> (index of element=w567:i32)  [unwired: 1 in]
        n259 = property on="교정값" class="Str"(error in=w573) -> (error out=w569:errorcluster, "Label.Text"=w572:string)  [unwired: 1 in, 1 out]
        n260 = Search 1D Array(1D array=w564, element=w572) -> (index of element=w566:i32)  [unwired: 1 in]
        n261 = case shown="기본" w576 {
          selector: w576 -> [_ w591]
          tunnel: w577 -> [_ w596]
          tunnel: w568 -> [_ w590]
          tunnel: w562 -> [_ w584]
          tunnel: w567 -> [_ w582]
          tunnel: w566 -> [_ w583]
          tunnel: w560 -> [_ w585]
          tunnel: w559 -> [_ w581]
          frame 0 {
          }
          frame Default {
            n262 = Decrement(x=w591) -> (x-1=w592:i32)
            n263 = Index Array(array=w596, index (col) #1=4 ("비활성화된 인덱스 (열)"), index (row) #2=w592) -> (element #1=w579:string[], element #2=w595:string[])  [unwired: 2 in]
            n264 = case shown="\"20414-0\"" w581 {
              tunnel: w595 -> [w617 w637 w664]
              tunnel: "교정점" -> [_ w635 w663]
              tunnel: w590 -> [_ w634 w662]
              tunnel: [w618 w638 w660] -> w589
              tunnel: "추가단위" -> [w597 w636 w656]
              tunnel: "명목값" -> [w599 _ w655]
              tunnel: "교정값" -> [w598 _ w654]
              tunnel: w585 -> [_ _ w653]
              tunnel: w584 -> [_ _ w652]
              tunnel: w583 -> [_ _ w651]
              tunnel: w582 -> [_ _ w650]
              tunnel: w579 -> [_ _ _]
              frame "20116-2" {
                w606 = dbl[] [1.0, 2.0, 5.0, 10.0, 20.0, 50.0, 100.0, 200.0, 500.0, 1000.0, 2000.0, 5000.0, 10000.0, 20000.0, 50000.0]
                n265 = case shown="\"N\"" w597 {
                  tunnel: [1.0 1e-06 0.001 1.0 1000.0 1000000.0 28.34952 453.5924 101.9716] -> w600
                  frame Default {
                  }
                  frame "μg" {
                  }
                  frame "mg" {
                  }
                  frame "g" {
                  }
                  frame "kg" {
                  }
                  frame "ton" {
                  }
                  frame "oz" {
                  }
                  frame "lb" {
                  }
                  frame "N" {
                  }
                }
                n266 = Fract/Exp String To Number(string=w598) -> (number=w602:dbl)  [unwired: 3 in, 1 out]
                n267 = Multiply(x=w602, y=w600) -> (x*y=w601:dbl)
                n268 = for {
                  tunnel: w601 -> [w633]
                  tunnel: w606 -> [w632] mode=indexing
                  tunnel: [w630] -> w607
                  i -> [w630]
                  stop <- w631 stop-if-true
                  n269 = Less?(x=w633, y=w632) -> (x < y?=w631:bool)
                }
                n270 = Decrement(x=w607) -> (x-1=w608:i32)
                n271 = Index Array(array=w606, index #1=w608) -> (element #1=w613:dbl, element #2=w614:dbl)  [unwired: 1 in]
                n272 = Add(x=w613, y=w614) -> (x+y=w609:dbl)
                n273 = Divide(x=w609, y=2.0) -> (x/y=w611:dbl)
                n274 = Greater Or Equal?(x=w611, y=w601) -> (x >= y?=w612:bool)
                n275 = Format Into String(format string="%#.6f" ("포맷 문자열"), w601) -> (resulting string=w603:string)  [unwired: 2 in, 1 out]
                n276 = Select(t=w613, s=w612, f=w614) -> (s? t:f=w616:dbl)
                n277 = Format Into String(format string="%.0f" ("포맷 문자열"), w616) -> (resulting string=w605:string)  [unwired: 2 in, 1 out]
                n278 = Replace Array Subset(array=w617, new element #1=w599, index #1=2 ("인덱스"), new element #2=w598, new element #3=w597, new element #4=w603, new element #5=w605, new element #6="g") -> (w618:string[])  [unwired: 5 in]
              }
              frame "20414-0" {
                n279 = Multiply(x=9.80665, y=0.9991026) -> (x*y=w645:dbl)
                n280 = call "Unit Conversion.vi"("환산단위"="kPa", "입력단위"=w636, "입력값"=w635) -> ("환산단위"=w640:string, "환산값 (DBL)"=w644:dbl, "환산값 (string)"=w639:string)  [unwired: 3 in, 3 out]
                n281 = Divide(x=w644, y=w645) -> (x/y=w646:dbl)
                n282 = Format Into String(format string="%.2f" ("포맷 문자열"), w646) -> (resulting string=w648:string)  [unwired: 2 in, 1 out]
                n283 = Replace Array Subset(array=w637, new element #1=w639, index #1=w634, new element #2=w640, new element #3=w648, index #3=2 ("인덱스")) -> (w638:string[])  [unwired: 1 in]
              }
              frame Default {
                n284 = case shown="기본" w662 {
                  selector: w662 -> [_ w707]
                  tunnel: w664 -> [w705 w709]
                  tunnel: w663 -> [_ w706]
                  tunnel: [w705 w708] -> w659
                  frame -1 {
                  }
                  frame Default {
                    n285 = case shown="기본" w706 {
                      selector: w706 -> [_ w711]
                      tunnel: w709 -> [w710 w714]
                      tunnel: [w710 w713] -> w708
                      tunnel: w707 -> [_ w712]
                      frame "" {
                      }
                      frame Default {
                        n286 = Replace Array Subset(array=w714, new element=w711, index=w712) -> (w713:string[])
                      }
                    }
                  }
                }
                n287 = case shown="기본" w652 {
                  selector: w652 -> [_ w697]
                  tunnel: w659 -> [w695 w699]
                  tunnel: w656 -> [_ w696]
                  tunnel: [w695 w698] -> w658
                  frame -1 {
                  }
                  frame Default {
                    n288 = case shown="기본" w696 {
                      selector: w696 -> [_ w701]
                      tunnel: w699 -> [w700 w704]
                      tunnel: [w700 w703] -> w698
                      tunnel: w697 -> [_ w702]
                      frame "" {
                      }
                      frame Default {
                        n289 = Replace Array Subset(array=w704, new element=w701, index=w702) -> (w703:string[])
                      }
                    }
                  }
                }
                n290 = case shown="기본" w653 {
                  selector: w653 -> [_ w687]
                  tunnel: w658 -> [w685 w689]
                  tunnel: w656 -> [_ w686]
                  tunnel: [w685 w688] -> w657
                  frame -1 {
                  }
                  frame Default {
                    n291 = case shown="기본" w686 {
                      selector: w686 -> [_ w691]
                      tunnel: w689 -> [w690 w694]
                      tunnel: [w690 w693] -> w688
                      tunnel: w687 -> [_ w692]
                      frame "" {
                      }
                      frame Default {
                        n292 = Replace Array Subset(array=w694, new element=w691, index=w692) -> (w693:string[])
                      }
                    }
                  }
                }
                n293 = case shown="기본" w650 {
                  selector: w650 -> [_ w677]
                  tunnel: w657 -> [w675 w679]
                  tunnel: w655 -> [_ w676]
                  tunnel: [w675 w678] -> w661
                  frame -1 {
                  }
                  frame Default {
                    n294 = case shown="기본" w676 {
                      selector: w676 -> [_ w681]
                      tunnel: w679 -> [w680 w684]
                      tunnel: [w680 w683] -> w678
                      tunnel: w677 -> [_ w682]
                      frame "" {
                      }
                      frame Default {
                        n295 = Replace Array Subset(array=w684, new element=w681, index=w682) -> (w683:string[])
                      }
                    }
                  }
                }
                n296 = case shown="기본" w651 {
                  selector: w651 -> [_ w667]
                  tunnel: w661 -> [w665 w669]
                  tunnel: w654 -> [_ w666]
                  tunnel: [w665 w668] -> w660
                  frame -1 {
                  }
                  frame Default {
                    n297 = case shown="기본" w666 {
                      selector: w666 -> [_ w671]
                      tunnel: w669 -> [w670 w674]
                      tunnel: [w670 w673] -> w668
                      tunnel: w667 -> [_ w672]
                      frame "" {
                      }
                      frame Default {
                        n298 = Replace Array Subset(array=w674, new element=w671, index=w672) -> (w673:string[])
                      }
                    }
                  }
                }
              }
            }
            n299 = Insert Into Array(array=w596, index (row)=w591, new element=w589) -> (w593:string[][])  [unwired: 1 in]
            n300 = local write "Proc"(w593) -> ()
          }
        }
      }
      frame "종료" {
      }
      frame "에러" {
        n301 = Variant To Data(error in=w721, type=errorcluster {"status"=FALSE, "code"=0, "source"=""} ("에러 출력"), Variant=w719) -> (data=w717:errorcluster, error out=w718:errorcluster)
        n302 = call <vilib>:"Simple Error Handler.vi"("error in (no error)"=w717) -> ()  [unwired: 4 in, 5 out]
      }
    }
  }
  n303 = Merge Errors(w16, w17) -> (w15:errorcluster)
  n304 = call <vilib>:"Simple Error Handler.vi"("error in (no error)"=w15) -> ("error out"=→"error out":errorcluster)  [unwired: 4 in, 4 out]
